vi "SRV_String to String Array.vi"(1 "Element Separator (,)":string=",", 7 "String":string, 12 "Trim Output Elements? (T)":bool=TRUE) -> (8 "String Array":string[](array[string]))   [LabVIEW 2014]
doc: "Separate String into an array of strings. The Element Separator is removed from the string elements.\n\n\nAuthor: Mike Schultz\n\n\nLogicPD, Inc\nwww.logicpd.com"
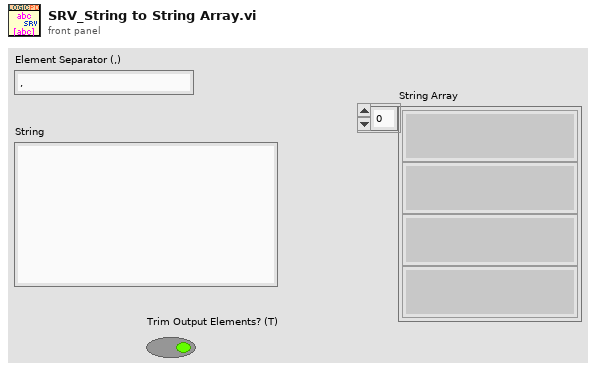
[diagram p1: front panel]
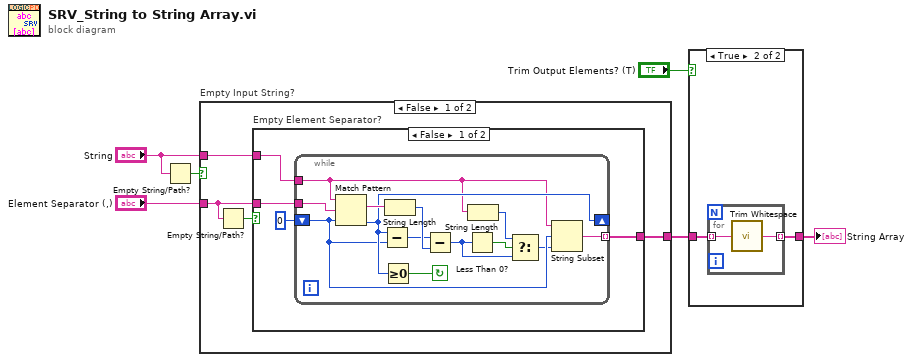
[diagram p0: block diagram]
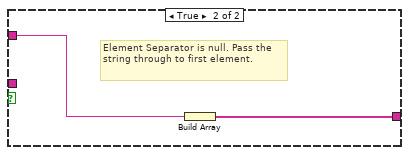
[diagram p3: hidden frame]
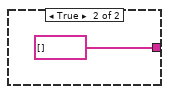
[diagram p4: hidden frame]
diagram:
  n1 = Empty String/Path?(string/path="String") -> (empty?=w6:bool)
  n2 = case "Empty Input String?" shown="False" w6 {
    tunnel: [w10 string[] []] -> w3
    tunnel: "Element Separator (,)" -> [w9 _]
    tunnel: "String" -> [w7 _]
    frame False {
      n3 = Empty String/Path?(string/path=w9) -> (empty?=w8:bool)
      n4 = case "Empty Element Separator?" shown="False" w8 {
        tunnel: [w14 w28] -> w10
        tunnel: w7 -> [w13 w29]
        tunnel: w9 -> [w12 _]
        frame False {
          n5 = while {
            tunnel: [w26] -> w14 mode=indexing
            tunnel: w12 -> [w15]
            tunnel: w13 -> [w19]
            shift-left: 0 -> [w21]
            shift-right: [w22] -> _
            stop <- w27 continue-if-true
            n6 = Match Pattern(string=w19, regular expression=w15, offset (0)=w21) -> (match substring=w25:string, offset past match=w22:i32)  [unwired: 2 out]
            n7 = Subtract(x=w22, y=w21) -> (x-y=w23:i32)
            n8 = Greater Or Equal To 0?(x=w22) -> (x >= 0?=w27:bool)
            n9 = String Length(string=w25) -> (length=w24:i32)
            n10 = Subtract(x=w23, y=w24) -> (x-y=w16:i32)
            n11 = Less Than 0?(x=w16) -> (x < 0?=w20:bool)
            n12 = String Length(string=w19) -> (length=w17:i32)
            n13 = Select(t=w17, s=w20, f=w16) -> (s? t:f=w18:i32)
            n14 = String Subset(string=w19, offset (0)=w21, length (rest)=w18) -> (substring=w26:string)
          }
        }
        frame True {
          # "Element Separator is null. Pass the string through to first element."
          n15 = Build Array(w29) -> (w28:string[])
        }
      }
    }
    frame True {
    }
  }
  n16 = case shown="True" "Trim Output Elements? (T)" {
    tunnel: w3 -> [w31 w33]
    tunnel: [w31 w32] -> w2
    frame False {
    }
    frame True {
      n17 = for {
        tunnel: w33 -> [w35] mode=indexing
        tunnel: [w34] -> w32 mode=indexing
        n18 = call <vilib>:"Trim Whitespace.vi"("string"=w35) -> ("trimmed string"=w34:string)  [unwired: 1 in]
      }
    }
  }
  "String Array" <- w2
